vi "Transitions.vi"(6 "State Loop Data in":T1, 11 "State in":refnum<class "State.lvclass">) -> (2 "Met Conditions":refnum<class "Condition.lvclass">[](array[class]), 3 "State out":refnum<class "State.lvclass">, 4 "State Loop Data":T1)   [LabVIEW 2023, in "VolatusSeq.lvlib" / "State.lvclass"]
uses:
  State.lvclass
  State Loop Data.ctl
  Iteration Actions/Iteration Actions.lvclass
  Variables/Variables.lvclass
  Command.ctl
  VolatusSeqConfig/Command Type.ctl
  messages/CmdDigital/Data.ctl
  messages/CmdAnalog/Data.ctl
  Send Type.ctl
  Sequence Time.ctl
  Condition/Condition.lvclass
  State.lvclass/State.ctl
  Transition/Transition.lvclass
  VolatusSeq.lvlib
  VolatusSeqConfig/VolatusSeqConfig.lvlib
  Volatus/MessageQ/MessageQ.lvclass
  messages/CmdDigital/CmdDigital.lvlib
  messages/CmdAnalog/CmdAnalog.lvlib
  lv-vecto/Vecto/Channel DBL/Channel DBL.lvclass
  Format String/Format String.lvclass
  VolatusSeqConfig/Debug Flags.ctl
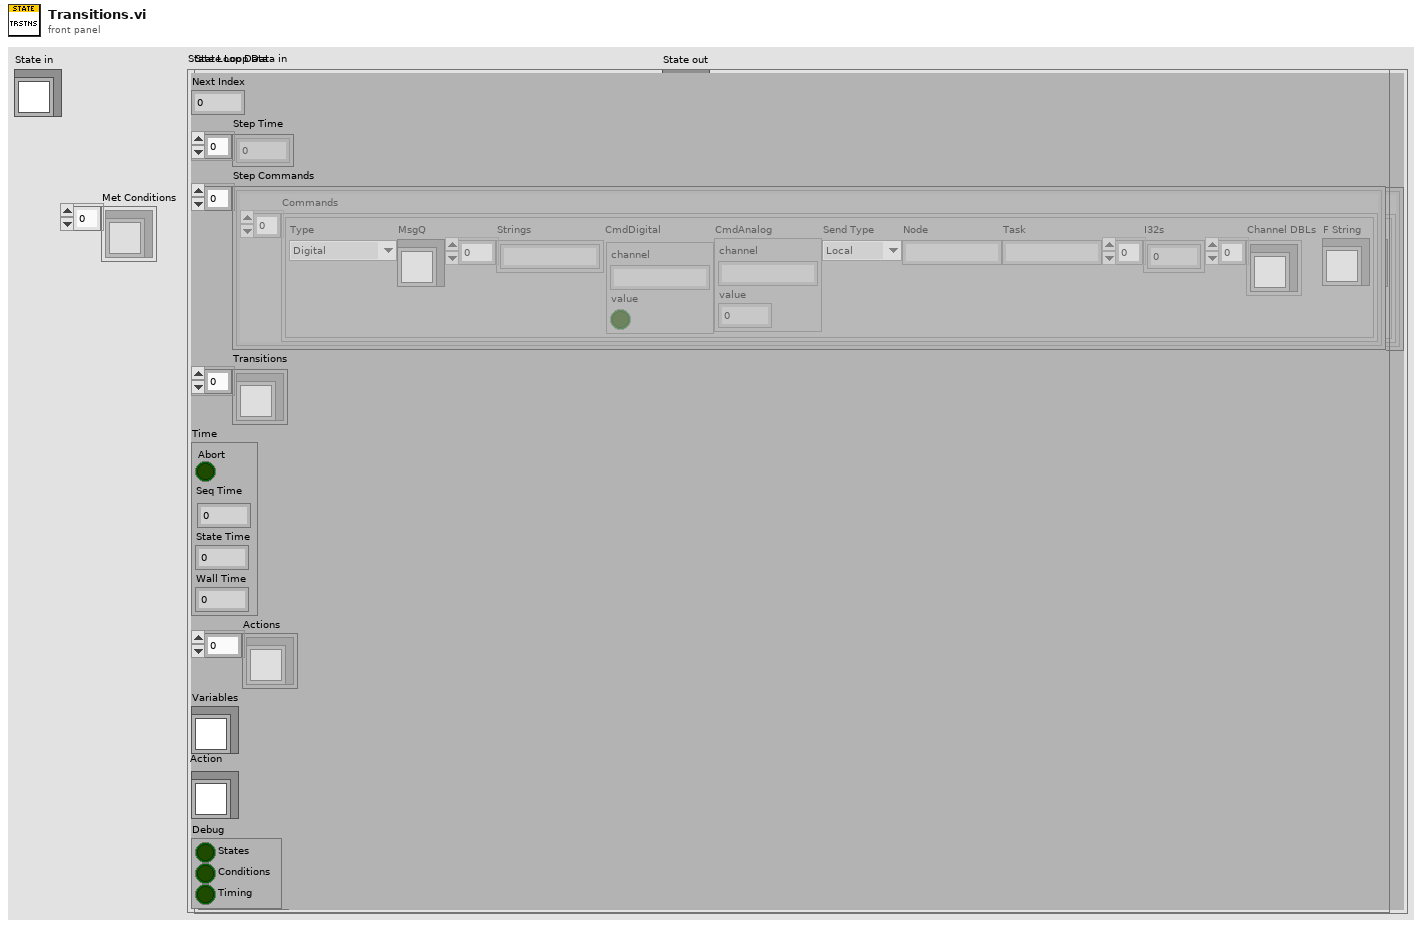
[diagram p1: front panel]
types:
  T1 = typedef "VolatusSeq.lvlib/State.lvclass/State Loop Data.ctl" = cluster{"Next Index":i32, "Step Time":dbl[], "Step Commands":cluster{"Commands":T2[]}[], "Transitions":refnum<class "Transition.lvclass">[], "Time":T7, "Actions":refnum<class "Iteration Actions.lvclass">[], "Variables":refnum<class "Variables.lvclass">, "Action":refnum<class "Iteration Actions.lvclass">, "Debug":T8}
  T2 = typedef "VolatusSeq.lvlib/Command.ctl" = cluster{"Type":T3, "MsgQ":refnum<class "MessageQ.lvclass">, "Strings":string[], "CmdDigital":T4, "CmdAnalog":T5, "Send Type":T6, "Node":string, "Task":string, "I32s":i32[], "Channel DBLs":refnum<class "Channel DBL.lvclass">[], "F String":refnum<class "Format String.lvclass">}
  T3 = typedef "VolatusSeqConfig.lvlib/Command Type.ctl" = enum16{"Digital", "Numeric", "Transition", "Stop", "StartLog", "StopLog", "Start", "Event", "Error", "HTTP", "ResetVar", "IncVar", "DecVar", "SaveVar", "LoadVar", "AddVar", "SubVar", "SetVar", "AddToVar"}
  T4 = typedef "CmdDigital.lvlib/Data.ctl" = cluster{"channel":string, "value":bool}
  T5 = typedef "CmdAnalog.lvlib/Data.ctl" = cluster{"channel":string, "value":dbl}
  T6 = typedef "VolatusSeq.lvlib/Send Type.ctl" = enum16{"Local", "Remote"}
  T7 = typedef "VolatusSeq.lvlib/Sequence Time.ctl" = cluster{"Abort":bool, "Seq Time":dbl, "State Time":dbl, "Wall Time":dbl}
  T8 = typedef "VolatusSeqConfig.lvlib/Debug Flags.ctl" = cluster{"States":bool, "Conditions":bool, "Timing":bool}
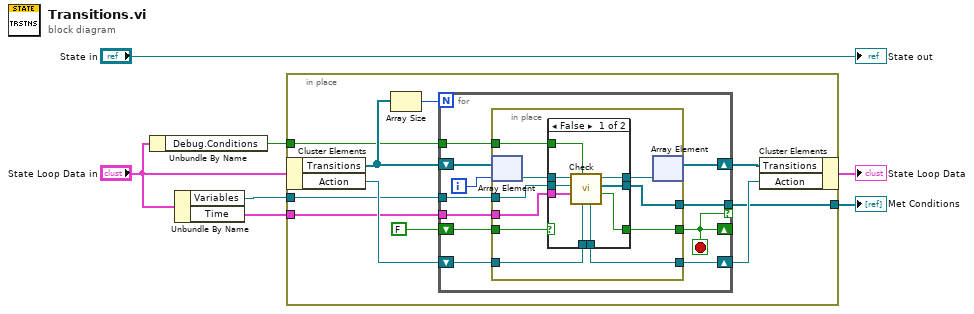
[diagram p0: block diagram]
diagram:
  n1 = Unbundle By Name("State Loop Data in") -> ("Debug.Conditions"=w2:bool)
  n2 = Unbundle By Name("State Loop Data in") -> ("Variables"=w1:refnum<class "Variables.lvclass">, "Time"=w5:T7)
  n3 = in-place {
    in-place-border: w5 -> [w14]
    in-place-border: [w10] -> w4
    in-place-border: w2 -> [w9]
    in-place-border: w1 -> [w8]
    n4 = in-place-cluster #1("State Loop Data in") -> ("Transitions"=w12:refnum<class "Transition.lvclass">[], "Action"=w17:refnum<class "Iteration Actions.lvclass">)
    n5 = Array Size(array=w12) -> (size(s)=w11:i32)
    n6 = for {
      N: w11 -> [_]
      shift-right: [w27] -> w15
      shift-left: w17 -> [w28]
      tunnel: w14 -> [w26]
      shift-right: [w20] -> _
      shift-left: FALSE -> [w25]
      shift-right: [w22] -> w16
      shift-left: w12 -> [w24]
      tunnel: [w21] -> w10 if=w20
      tunnel: w9 -> [w19]
      tunnel: w8 -> [w18]
      i -> [w23]
      stop <- w20 stop-if-true
      n7 = in-place {
        in-place-border: w28 -> [w38]
        in-place-border: [w37] -> w27
        in-place-border: w26 -> [w36]
        in-place-border: w25 -> [w35]
        in-place-border: [w34] -> w20
        in-place-border: [w31] -> w21
        in-place-border: w19 -> [w30]
        in-place-border: w18 -> [w29]
        n8 = in-place-array #2(w24, w23) -> (w33:refnum<class "Transition.lvclass">)
        n9 = case shown="False" w35 {
          selector: w35 -> [_ w48]
          tunnel: w33 -> [w47 w49]
          tunnel: w38 -> [w46 w50]
          tunnel: [w45 w49] -> w32
          tunnel: [w44 w50] -> w37
          tunnel: w29 -> [w43 _]
          tunnel: w36 -> [w42 _]
          tunnel: [w41 w48] -> w34
          tunnel: [w40 _] -> w31
          tunnel: w30 -> [w39 _]
          frame False {
            n10 = call "Check.vi"("Actions In"=w46, "Report Conditions"=w39, "Sequence Time"=w42, "Variables"=w43, "Transition in"=w47) -> ("Triggered"=w41:bool, "Met Conditions"=w40:refnum<class "Condition.lvclass">[], "Transition out"=w45:refnum<class "Transition.lvclass">, "Actions"=w44:refnum<class "Iteration Actions.lvclass">)  [unwired: 3 in]
          }
          frame True {
          }
        }
        n11 = in-place-array #2(w32) -> (w22:refnum<class "Transition.lvclass">[])  [unwired: 1 out]
      }
    }
    n12 = in-place-cluster #1("Transitions"=w16, "Action"=w15) -> (→"State Loop Data":T1)
  }
  "Met Conditions" <- w4
  "State out" <- "State in"
